vi "ParseDataSendParameters.vi"(8 "error in (no error)":errorcluster, 11 "body":variant) -> (0 "error out":errorcluster, 3 "data send parameters":T1)   [LabVIEW 2017, in "ServerComm.lvlib"]
uses:
  <vilib>/addons/InsightCM/Devices/Shared/Common/ServerComm/ServerComm.lvlib
  <vilib>/addons/InsightCM/Devices/Shared/Common/ServerComm/controls/DataSendParameters.ctl
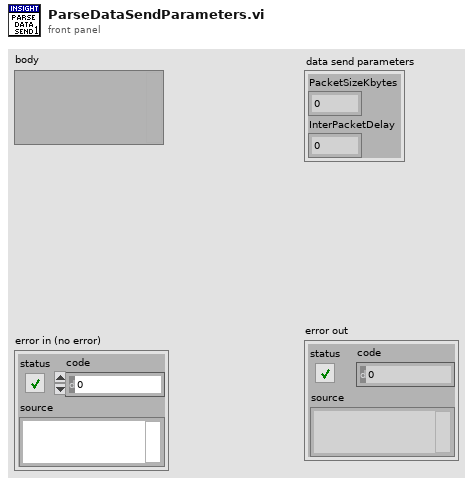
[diagram p1: front panel]
types:
  T1 = typedef "ServerComm.lvlib/DataSendParameters.ctl" = cluster{"PacketSizeKbytes":i32, "InterPacketDelay":i32}
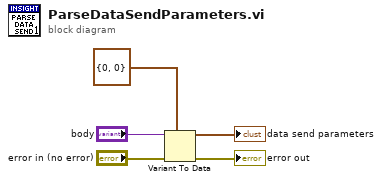
[diagram p0: block diagram]
diagram:
  n1 = Variant To Data(error in="error in (no error)", type=T1 {"PacketSizeKbytes"=0, "InterPacketDelay"=0} ("DataSendParameters"), Variant="body") -> (data=→"data send parameters":T1, error out=→"error out":errorcluster)
